vi "APIBIasDiffUpdateIODOCS.vi"(8 "Error In":errorcluster, 11 "Data":variant) -> (0 "Error Out":errorcluster)   [LabVIEW 2023, in "QSM - IODocs.lvlib"]
uses:
  QSM - IODocs.lvlib
  Controls/Message Queue Element Position.ctl
  Controls/State Machine Message.ctl
  SubVIs/Enqueue Message (Single).vi
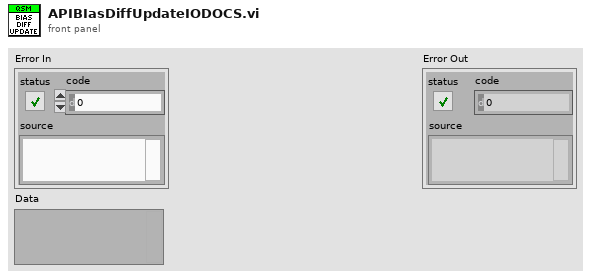
[diagram p1: front panel]
types:
  T1 = typedef "QSM - IODocs.lvlib/State Machine Message.ctl" = enum16{"Initialize", "BIAS ZERO", "DIFF ZERO", "DIFF TOGGLE", "UpdateAIO", "UpdateBiasDiff", "GxValsUpdate", "OffsetGainUpdate", "APIAIOUpdate", "APIGridValsUpdate", "APIBiasDiffUpdate", "Handle Error", "Exit"}
  T2 = typedef "QSM - IODocs.lvlib/Message Queue Element Position.ctl" = enum16{"Front", "Back"}
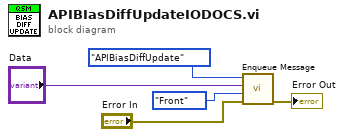
[diagram p0: block diagram]
diagram:
  n1 = call-poly "Enqueue Message.vi"("Error In"="Error In", "Message Position"=Message_Queue_Element_Position."Front", "Data"="Data", "State Machine Message"=State_Machine_Message."APIBiasDiffUpdate") -> ("Error Out"=→"Error Out":errorcluster)  [unwired: 7 in]
